vi "pf_Get_Error_msg.vi"(8 "error in (no error)":errorcluster, 10 "iPort":i32, 11 "error code":i32) -> (0 "error out":errorcluster, 3 "pf_Error_msg":string)   [LabVIEW 2012, in "Photonfocus_Toolkit.lvlib"]
uses:
  <userlib>/Photonfocus Toolkit/Photonfocus_Toolkit.lvlib
  <userlib>/Photonfocus Toolkit/_Private/Controls/pf_Toolkit_Error_Type.ctl
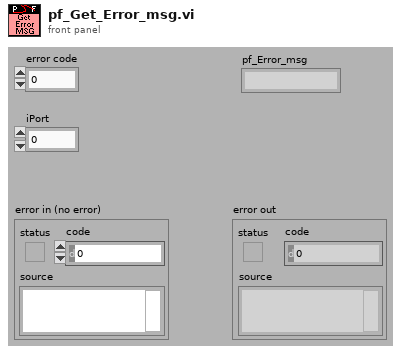
[diagram p1: front panel]
types:
  T1 = typedef "Photonfocus_Toolkit.lvlib/pf_Toolkit_Error_Type.ctl" = enum16{"PF Toolkit_Generic Error", "PF Toolkit_PFConfig Error"}
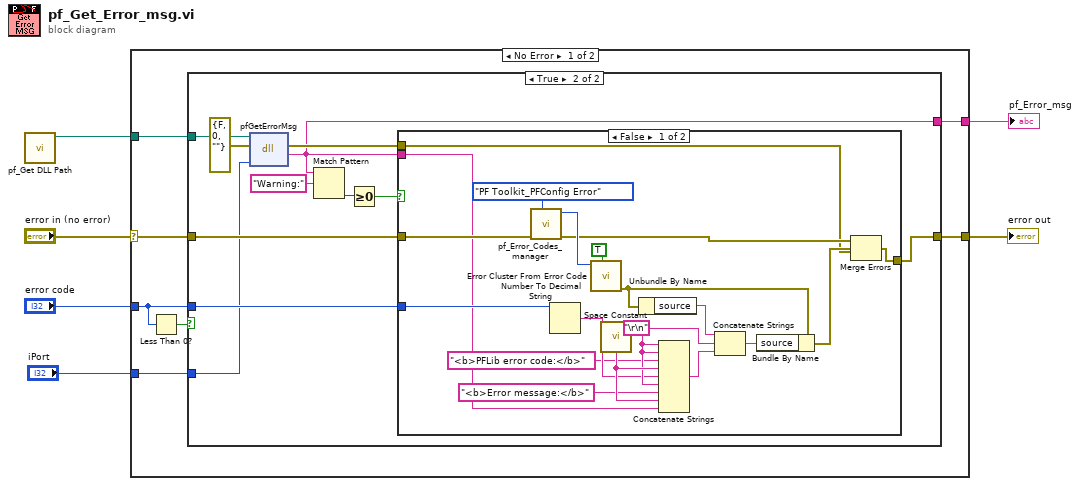
[diagram p0: block diagram]
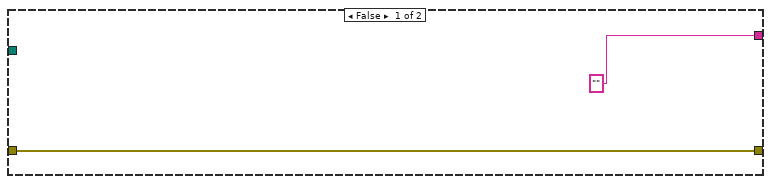
[diagram p2: hidden frame]
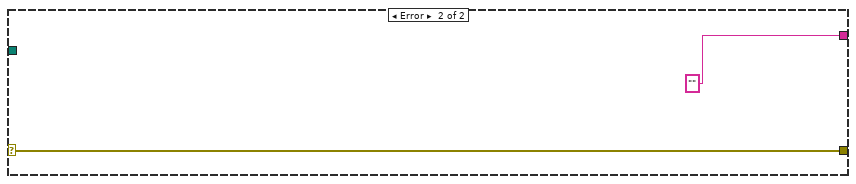
[diagram p4: hidden frame]
diagram:
  n1 = call <userlib>:"pf_Get DLL Path.vi"() -> ("DLL path"=w4:path)  [unwired: 1 in, 10 out]
  n2 = case shown="No Error" "error in (no error)" {
    selector: "error in (no error)" -> [w13 w48]
    tunnel: [w12 w48] -> w6
    tunnel: "error code" -> [w9 _]
    tunnel: w4 -> [w11 _]
    tunnel: [w10 "" ("return type")] -> w3
    tunnel: "iPort" -> [w7 _]
    frame No Error {
      n3 = Less Than 0?(x=w9) -> (x < 0?=w8:bool)
      n4 = case shown="True" w8 {
        tunnel: w13 -> [w15 w25]
        tunnel: w9 -> [_ w23]
        tunnel: [w15 w24] -> w12
        tunnel: w11 -> [_ w26]
        tunnel: ["" ("return type") w20] -> w10
        tunnel: w7 -> [_ w16]
        frame False {
        }
        frame True {
          n5 = dll-call lib="S:/Progetti/Photonfocus/Codice/DEV/PFConfig_lvlib/PFConfig.*" fn="pfGetErrorMsg"(path in=w26, error in=errorcluster {"status"=FALSE, "code"=0, "source"=""} ("error in (no error)"), "iPort"=w16) -> (error out=w22:errorcluster, "return type"=w20:string)  [unwired: 1 in, 2 out]
          n6 = Match Pattern(string=w20, regular expression="Warning:") -> (offset past match=w18:i32)  [unwired: 4 out]
          n7 = Greater Or Equal To 0?(x=w18) -> (x >= 0?=w17:bool)
          n8 = case shown="False" w17 {
            tunnel: w25 -> [w44 w46]
            tunnel: [w30 w46] -> w24
            tunnel: w23 -> [w29 _]
            tunnel: w22 -> [w28 _]
            tunnel: w20 -> [w27 _]
            frame False {
              w40 = "\r\n"
              n9 = call <userlib>:"pf_Error_Codes_manager.vi"("pf Error Type"=pf_Toolkit_Error_Type."PF Toolkit_PFConfig Error", "error in (no error)"=w44) -> ("error out"=w34:errorcluster, "pf Error Code"=w42:i32)  [unwired: 8 out]
              n10 = Number To Decimal String(number=w29) -> (decimal integer string=w36:string)  [unwired: 1 out]
              n11 = call <vilib>:"Error Cluster From Error Code.vi"("show call chain? (False)"=TRUE, "error code (0)"=w42) -> ("error out"=w33:errorcluster)  [unwired: 1 in, 6 out]
              n12 = call <vilib>:"Space Constant.vi"() -> ("String"=w41:string)
              n13 = Unbundle By Name(w33) -> ("source"=w38:string)
              n14 = Concatenate Strings(w40, w40, "<b>PFLib error code:</b>" ("string"), w41, w36, w40, "<b>Error message:</b>" ("string"), w41, w27) -> (w37:string)
              n15 = Concatenate Strings(w38, w40, w37) -> (w32:string)
              n16 = Bundle By Name(cluster=w33, "source"=w32) -> (w31:errorcluster)
              n17 = Merge Errors(w34, w31, w28) -> (w30:errorcluster)
            }
            frame True {
            }
          }
        }
      }
    }
    frame Error {
    }
  }
  "error out" <- w6
  "pf_Error_msg" <- w3
